vi "Specify_Path.vi"(5 "Path_Enum":enum16{"Find_Path", "Get_Path"}(ring)=enum."Get_Path", 11 "error in (no error)":errorcluster) -> (2 "Application Directory":path, 3 "stripped path":path, 4 "Configurations":path, 6 "DATA":path, 8 "Modules path":path, 10 "Settings":path, 14 "path":path, 15 "error out":errorcluster)   [LabVIEW 2024, in "Launcher_DTU.lvlib"]
uses:
  Launcher_DTU.lvlib
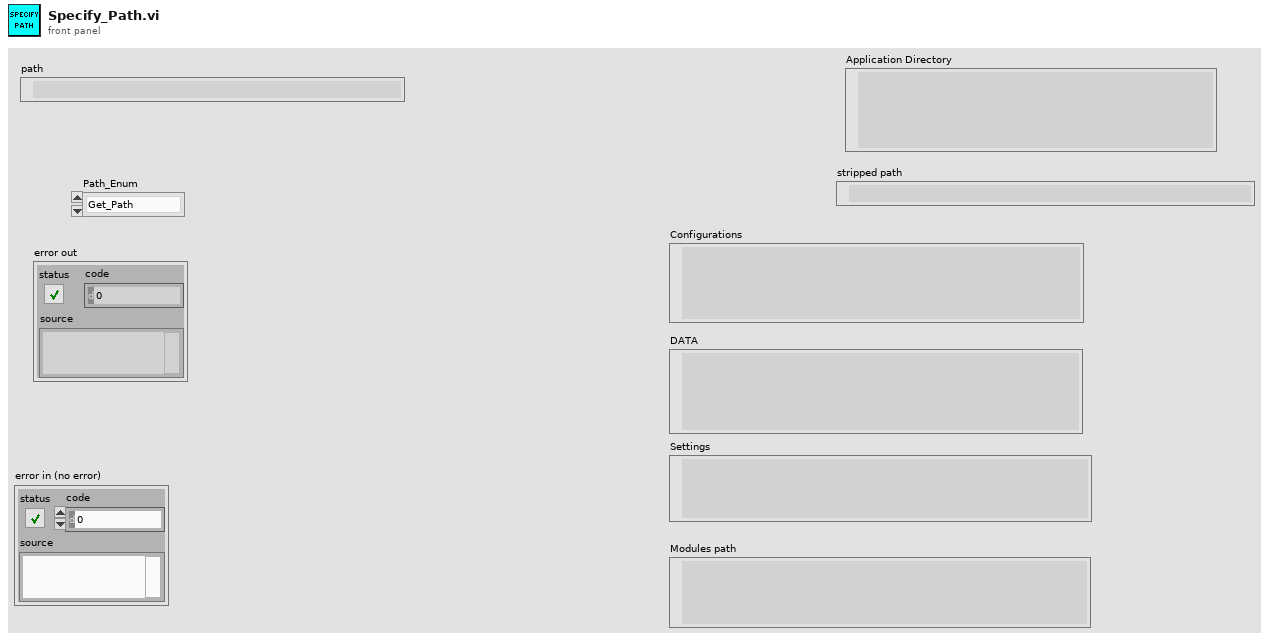
[diagram p1: front panel]
types:
  T1 = enum32{"invalid app kind", "Development System", "Run Time System", "Student Edition", "Embedded LabVIEW", "Evaluation", "Custom"}
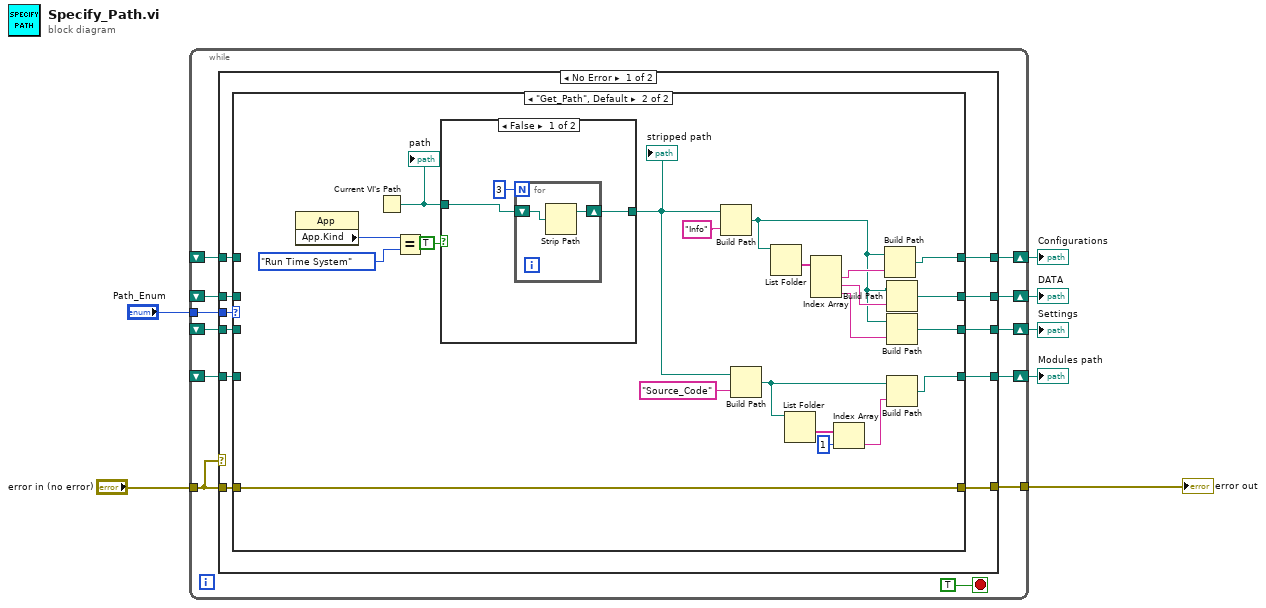
[diagram p0: block diagram]
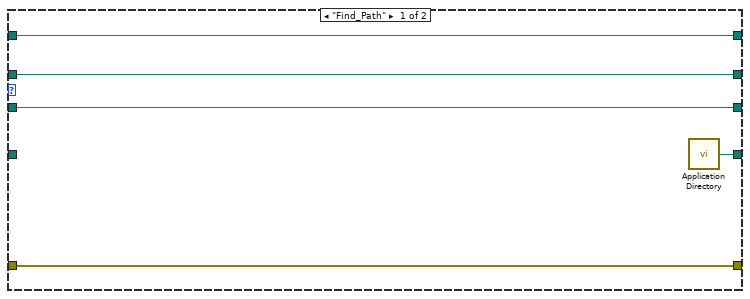
[diagram p2: hidden frame]
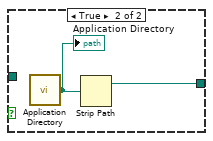
[diagram p3: hidden frame]
diagram:
  n1 = while {
    tunnel: "error in (no error)" -> [w18]
    tunnel: [w17] -> w6
    tunnel: "Path_Enum" -> [w16]
    shift-right: [w15] -> w4
    shift-left: _ -> [w13]
    shift-right: [w14] -> w3
    shift-left: _ -> [w12]
    shift-right: [w11] -> w2
    shift-left: _ -> [w10]
    shift-right: [w9] -> w1
    shift-left: _ -> [w8]
    stop <- TRUE stop-if-true
    n2 = case shown="No Error" w18 {
      tunnel: w18 -> [w30 w64]
      tunnel: [w29 w64] -> w17
      tunnel: w16 -> [w28 _]
      tunnel: [w27 _] -> w15
      tunnel: [w26 _] -> w14
      tunnel: w13 -> [w25 _]
      tunnel: w12 -> [w24 _]
      tunnel: [w23 _] -> w11
      tunnel: w10 -> [w22 _]
      tunnel: [w21 _] -> w9
      tunnel: w8 -> [w20 _]
      frame No Error {
        n3 = case shown="\"Get_Path\", Default" w28 {
          tunnel: w30 -> [w35 w56]
          tunnel: [w35 w56] -> w29
          tunnel: [w34 w48] -> w27
          tunnel: [w33 w47] -> w26
          tunnel: w25 -> [w34 _]
          tunnel: w24 -> [w33 _]
          tunnel: [w31 w38] -> w23
          tunnel: w22 -> [_ _]
          tunnel: [w32 w44] -> w21
          tunnel: w20 -> [w32 _]
          frame "Find_Path" {
            n4 = call <vilib>:"Application Directory.vi"() -> ("Application Directory"=w31:path)
          }
          frame "Get_Path", Default {
            n5 = property class="App"() -> ("App.Kind"=w55:T1)  [unwired: 2 in, 2 out]
            n6 = Current VI's Path() -> (path=w53:path)
            "path" <- w53
            n7 = Equal?(x=w55, y=T1."Run Time System" ("Application:Kind")) -> ()  [unwired: 1 out]
            n8 = case shown="False" TRUE {
              tunnel: w53 -> [w59 _]
              tunnel: [w57 w63] -> w41
              frame False {
                n9 = for {
                  N: 3 -> [_]
                  shift-right: [w60] -> w57
                  shift-left: w59 -> [w61]
                  n10 = Strip Path(path=w61) -> (stripped path=w60:path)  [unwired: 1 out]
                }
              }
              frame True {
                n11 = call <vilib>:"Application Directory.vi"() -> ("Application Directory"=w62:path)
                "Application Directory" <- w62
                n12 = Strip Path(path=w62) -> (stripped path=w63:path)  [unwired: 1 out]
              }
            }
            "stripped path" <- w41
            n13 = Build Path(base path=w41, name or relative path="Info") -> (appended path=w45:path)
            n14 = Build Path(base path=w41, name or relative path="Source_Code") -> (appended path=w39:path)
            n15 = List Folder(path=w45) -> (folder names=w51:string[])  [unwired: 3 in, 3 out]
            n16 = List Folder(path=w39) -> (folder names=w40:string[])  [unwired: 3 in, 3 out]
            n17 = Index Array(array=w51) -> (element #1=w50:string, element #2=w49:string, element #3=w46:string)  [unwired: 3 in]
            n18 = Index Array(array=w40, index=1) -> (element=w36:string)
            n19 = Build Path(base path=w45, name or relative path=w50) -> (appended path=w48:path)
            n20 = Build Path(base path=w45, name or relative path=w49) -> (appended path=w47:path)
            n21 = Build Path(base path=w45, name or relative path=w46) -> (appended path=w44:path)
            n22 = Build Path(base path=w39, name or relative path=w36) -> (appended path=w38:path)
          }
        }
      }
      frame Error {
      }
    }
  }
  "error out" <- w6
  "Configurations" <- w4
  "DATA" <- w3
  "Modules path" <- w2
  "Settings" <- w1
